vi "DIO 2-bit.vi"(0 "DIO0 Refnum":refnum<k21>, 1 "DIO1 Refnum":refnum<k21>, 2 "OUT 1:0":fxp<+,2,2> format="%b", 3 "DIR 1:0 2":fxp<+,2,2> format="%b") -> (10 "IN 1:0":fxp<+,2,2> format="%b")   [LabVIEW 2019]
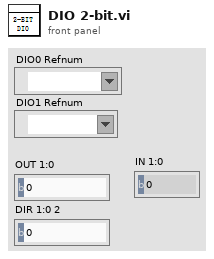
[diagram p1: front panel]
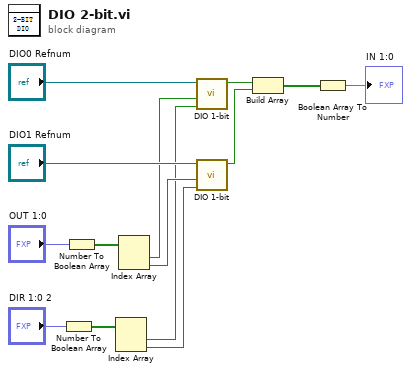
[diagram p0: block diagram]
diagram:
  n1 = Number To Boolean Array(number="DIR 1:0 2") -> (Boolean array=w10:bool[])
  n2 = Number To Boolean Array(number="OUT 1:0") -> (Boolean array=w11:bool[])
  n3 = Index Array(array=w10) -> (element #1=w6:bool, element #2=w5:bool)  [unwired: 2 in]
  n4 = Index Array(array=w11) -> (element #1=w8:bool, element #2=w7:bool)  [unwired: 2 in]
  n5 = call "DIO 1-bit.vi"("DIR"=w6, "OUT"=w8, "DIO Refnum"="DIO0 Refnum") -> ("IN"=w4:bool)  [unwired: 8 in]
  n6 = call "DIO 1-bit.vi"("DIR"=w5, "OUT"=w7, "DIO Refnum"="DIO1 Refnum") -> ("IN"=w3:bool)  [unwired: 8 in]
  n7 = Build Array(w4, w3) -> (w2:bool[])
  n8 = Boolean Array To Number(Boolean array=w2) -> (number=→"IN 1:0":fxp<+,2,2>)
